vi "My Launcher.vi"() -> ()   [LabVIEW 2018]
panel:
  in  "stop":bool
  out "error out":errorcluster
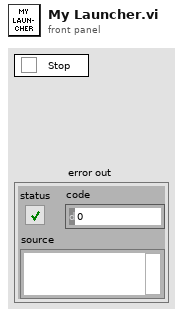
[diagram p1: front panel]
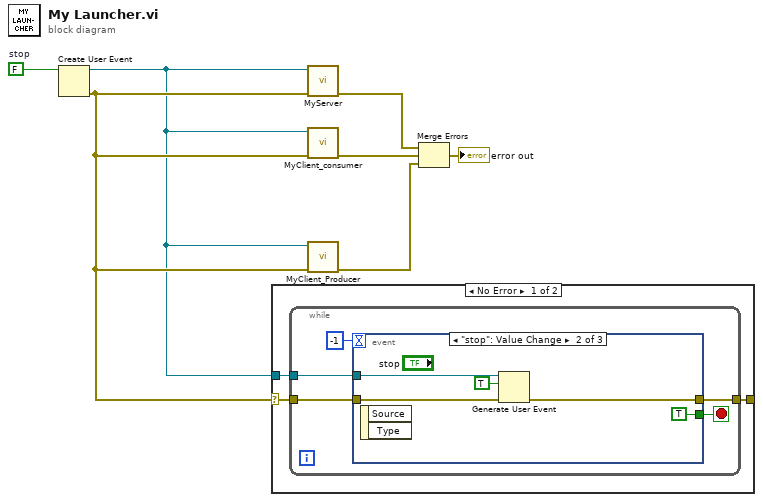
[diagram p0: block diagram]
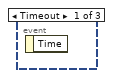
[diagram p2: hidden frame]
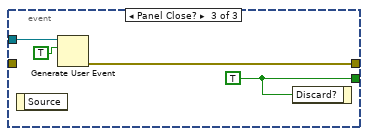
[diagram p3: hidden frame]
diagram:
  w7 = FALSE  # stop
  n1 = Create User Event(user event datatype=w7) -> (user event=w1:refnum<user-event>, error out=w2:errorcluster)  [unwired: 1 in]
  n2 = case shown="No Error" w2 {
    selector: w2 -> [w9 w25]
    tunnel: [w10 w25] -> _
    tunnel: w1 -> [w8 _]
    frame No Error {
      n3 = while {
        tunnel: [w13] -> w10
        tunnel: w9 -> [w12]
        tunnel: w8 -> [w11]
        stop <- w14 stop-if-true
        n4 = event shown="[1] \"stop\": Value Change" {
          selector: _ -> [_ _ _]
          dyn-events: _ -> [_ _ _]
          timeout: -1 -> [_ _ _]
          tunnel: [_ TRUE ("Discard?") w24] -> w14
          tunnel: [_ w17 w22] -> w13
          tunnel: w12 -> [_ w18 _]
          tunnel: w11 -> [_ w16 w21]
          event Timeout {
            n5 = event-data() -> ()  [unwired: 1 in, 1 out]
          }
          event "stop": Value Change {
            n6 = event-data() -> ()  [unwired: 1 in, 2 out]
            n7 = Generate User Event(user event=w16, event data cluster=TRUE ("event data"), error in=w18) -> (error out=w17:errorcluster)  [unwired: 1 in, 1 out]
          }
          event Panel Close? {
            w24 = TRUE ("Discard?")
            n8 = event-data() -> ()  [unwired: 1 in, 1 out]
            n9 = Generate User Event(user event=w21, event data cluster=TRUE ("event data")) -> (error out=w22:errorcluster)  [unwired: 2 in, 1 out]
            n10 = event-data("Discard?"=w24) -> ()  [unwired: 1 in, 1 out]
          }
        }
      }
    }
    frame Error {
    }
  }
  n11 = call "MyServer.vi"("error in (no error)"=w2, "Stop event"=w1) -> ("error server"=w6:errorcluster)  [unwired: 9 in]
  n12 = call "MyClient_consumer.vi"("error in (no error)"=w2, "Stop event"=w1) -> ("error client"=w5:errorcluster)  [unwired: 9 in]
  n13 = call "MyClient_Producer.vi"("error in (no error)"=w2, "Stop event"=w1) -> ("error client source"=w4:errorcluster)  [unwired: 9 in]
  n14 = Merge Errors(w6, w5, w4) -> (→"error out":errorcluster)
